vi "write Tx Rx.vi"(6 "length":u16, 7 "address":u16, 9 "id":u8, 10 "protocol_version":i32, 11 "port_num":i32) -> ()   [LabVIEW 2016, in "dxl_x86_c.lvlib"]
doc: "WINDECLSPEC void writeTxRx (int port_num, int protocol_version, uint8_t id, uint16_t address, uint16_t length);"
uses:
  dxl_x86_c.lvlib
  dxl_x86_c.dll
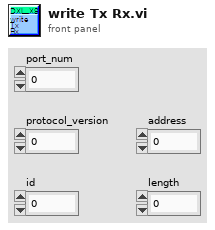
[diagram p1: front panel]
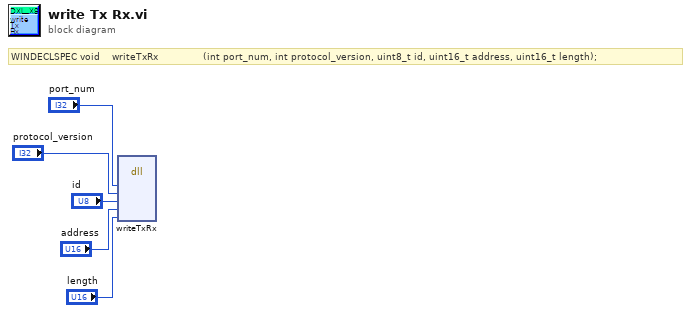
[diagram p0: block diagram]
diagram:
  # "WINDECLSPEC void    writeTxRx               (int port_num, int protocol_version, uint8_t id, uint16_t address, uint16_t length);"
  n1 = dll-call lib="C:/Users/Platform/Desktop/DynamixelSDK/labview/dxl_x86_c.lvlib/dxl_x86_c.*" fn="writeTxRx"("port_num"="port_num", "protocol_version"="protocol_version", "id"="id", "address"="address", "length"="length") -> ()  [unwired: 9 in, 2 out]
